vi "GW_update_id.vi"(5 "NULL: workplace_id":i16=-1, 7 "Set null":bool=TRUE, 8 "error in (no error)":errorcluster, 9 "glue_data_id":string="123", 10 "id":i16=5, 11 "DBlink":string="Driver={ODBC Driver 17 for SQL Server};Server=localhost\\SQLEXPRESS;Database=ZDX201;UID=labview;PWD=Dsa@54137926") -> (0 "error out":errorcluster)   [LabVIEW 2019]
uses:
  <vilib>/addons/database/Connection.llb/DB Tools Open Connec (String).vi
  <vilib>/addons/database/Connection.llb/Conn Execute.vi
  <vilib>/addons/database/Recordset.llb/Rec Fetch Recordset Data (R).vi
  <vilib>/addons/database/Recordset.llb/Rec Destroy - Connection.vi
  <vilib>/addons/database/_DB Variant To Data/Database Variant To Data.xnode
  <vilib>/addons/database/NI_Database_API.lvlib
panel:
  out "[glue_workspace]":cluster{"glue_data_id":string}[](array[cluster])
  out "查詢結果":string="Update [workplace_data] \nset  \n[barcode A] = NULL       \n  ,[barcode B] = NULL\n \n  where [workplace_name_id]= -1"
  out "Command":string="where [workplace_name_id]= 5"
  out "update value":T1={"glue_data_id"="123", "update time"=timestamp(3738130170.8632746 s since 1904-01-01)} {"update time" format="%<%.0X %x>T"}
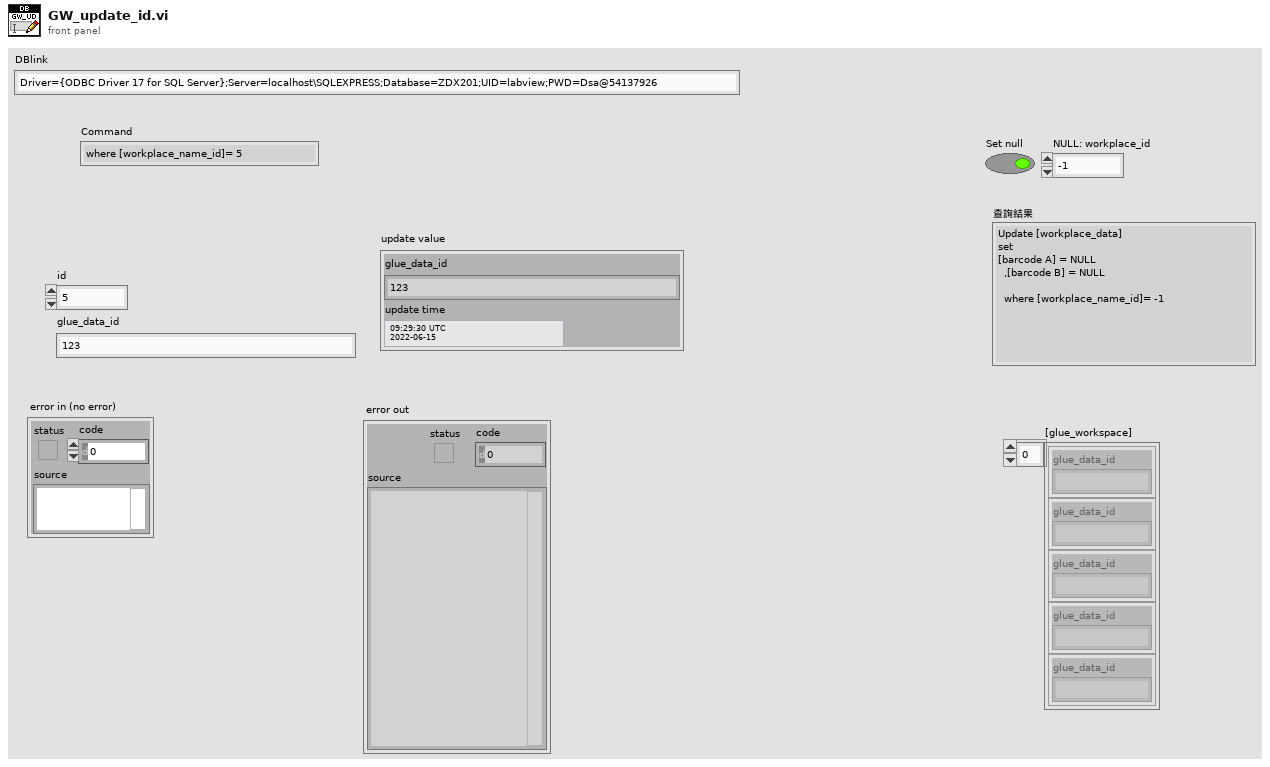
[diagram p1: front panel]
types:
  T1 = cluster{"glue_data_id":string, "update time":timestamp}
  T2 = typedef "NI_Database_API.lvlib/Conn ObjectReference.ctl" = refnum<k1>
  T3 = typedef "NI_Database_API.lvlib/Rec ObjectReference.ctl" = refnum<k1>
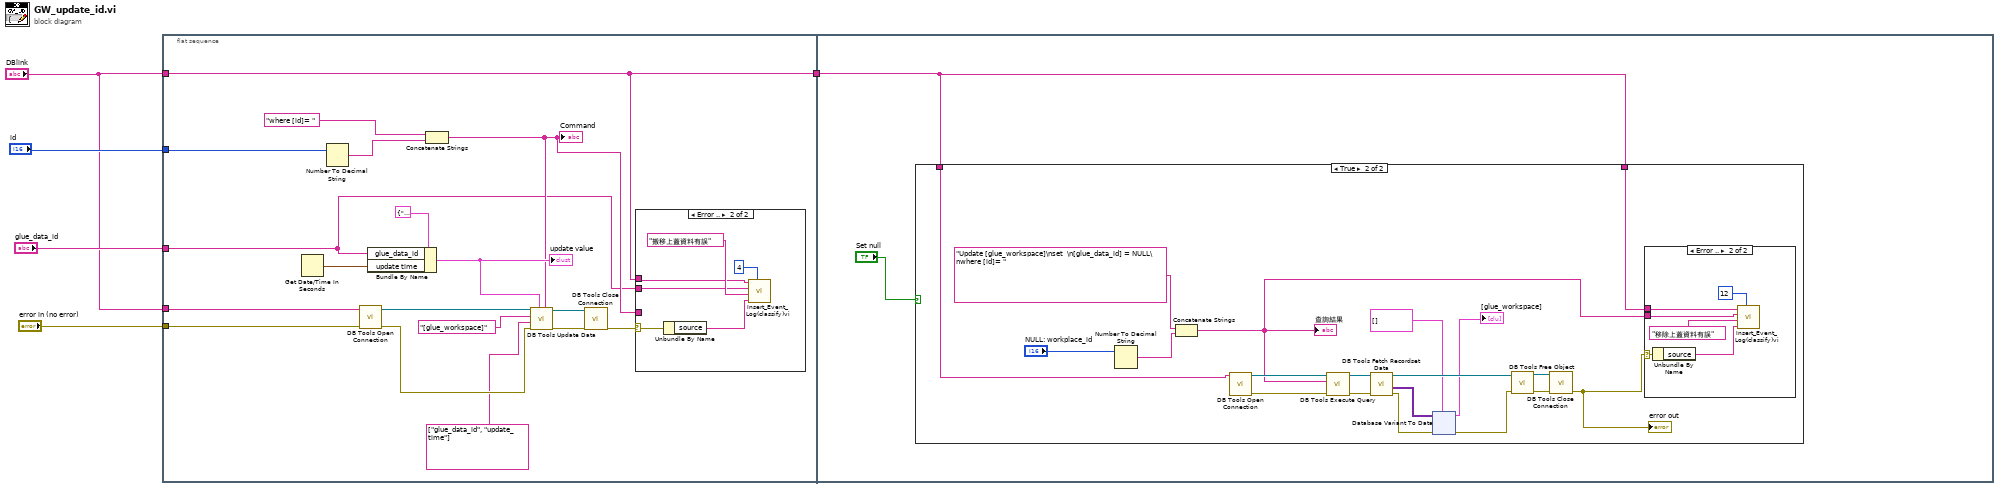
[diagram p0: block diagram]
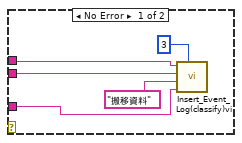
[diagram p2: hidden frame]
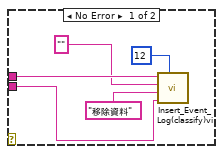
[diagram p4: hidden frame]
diagram:
  n1 = flat-sequence {
    tunnel: "error in (no error)" -> [w23]
    tunnel: "id" -> [w16]
    tunnel: "glue_data_id" -> [w6]
    tunnel: "DBlink" -> [w9]
    tunnel: "DBlink" -> [w7]
    tunnel: [w7] -> w1
    tunnel: w1 -> [w35]
    frame #0 {
      n2 = Get Date/Time In Seconds() -> (seconds since 1Jan1904=w15:timestamp)
      n3 = Number To Decimal String(number=w16) -> (decimal integer string=w13:string)  [unwired: 1 in]
      n4 = call-poly <vilib>:"DB Tools Open Connection.vi"("error in (no error)"=w23, "connection information"=w9) -> ("error out"=w21:errorcluster, "connection reference"=w19:T2)  [unwired: 6 in]
      n5 = Bundle By Name(cluster=T1 {"glue_data_id"="", "update time"=timestamp(0 s since 1904-01-01)} ("update value"), "glue_data_id"=w6, "update time"=w15) -> (w11:T1)
      "update value" <- w11
      n6 = Concatenate Strings("where [id]= ", w13) -> (w8:string)
      "Command" <- w8
      n7 = call <vilib>:"DB Tools Update Data.vi"("condition"=w8, "data"=w11, "error in (no error)"=w21, "columns"=string[] ["glue_data_id", "update_time"], "table"="[glue_workspace]", "connection reference"=w19) -> ("error out"=w22:errorcluster, "connection reference out"=w20:T2)  [unwired: 4 in]
      n8 = call <vilib>:"DB Tools Close Connection.vi"("error in (no error)"=w22, "connection reference"=w20) -> ("error out"=w10:errorcluster)  [unwired: 5 in]
      n9 = case shown="Error .." w10 {
        selector: w10 -> [_ w32]
        tunnel: w8 -> [w25 _]
        tunnel: w7 -> [w26 w30]
        tunnel: w6 -> [w24 w29]
        frame No Error {
          n10 = call "Insert_Event_Log(classify)vi.vi"("classify"=i16 3, "data"=w25, "message"="搬移資料", "id"=w24, "DBlink"=w26) -> ()  [unwired: 6 in, 1 out]
        }
        frame Error {
          n11 = Unbundle By Name(w32) -> ("source"=w31:string)
          n12 = call "Insert_Event_Log(classify)vi.vi"("classify"=i16 4, "data"=w31, "message"="搬移上蓋資料有誤", "id"=w29, "DBlink"=w30) -> ()  [unwired: 6 in, 1 out]
        }
      }
    }
    frame #1 {
      n13 = case shown="True" "Set null" {
        tunnel: w35 -> [_ w39]
        tunnel: w35 -> [_ w38]
        frame False {
        }
        frame True {
          n14 = Number To Decimal String(number="NULL: workplace_id") -> (decimal integer string=w55:string)  [unwired: 1 in]
          n15 = Concatenate Strings("Update [glue_workspace]\nset  \n[glue_data_id] = NULL\nwhere [id]= ", w55) -> (w37:string)
          "查詢結果" <- w37
          n16 = call-poly <vilib>:"DB Tools Open Connection.vi"("connection information"=w39) -> ("error out"=w44:errorcluster, "connection reference"=w45:T2)  [unwired: 7 in]
          n17 = call-poly <vilib>:"DB Tools Execute Query.vi"("error in (no error)"=w44, "SQL query"=w37, "connection reference"=w45) -> ("error out"=w47:errorcluster, "recordset reference"=w46:T3)  [unwired: 5 in]
          n18 = call-poly <vilib>:"DB Tools Fetch Recordset Data.vi"("error in (no error)"=w47, "recordset reference"=w46) -> ("error out"=w52:errorcluster, "recordset data"=w53:variant[][], "recordset reference out"=w51:T3)  [unwired: 3 in]
          n19 = xnode "Database Variant To Data"("database variant"=w53, "error in (no error)"=w52, "type"=cluster{"glue_data_id":string}[] [] ("Workplace: assemble")) -> ("data"=→"[glue_workspace]":cluster{"條碼B":string}[], "error out"=w50:errorcluster)
          n20 = call-poly <vilib>:"DB Tools Free Object.vi"("error in (no error)"=w50, "recordset reference"=w51) -> ("error out"=w49:errorcluster, "connection reference"=w48:T2)  [unwired: 8 in]
          n21 = call <vilib>:"DB Tools Close Connection.vi"("error in (no error)"=w49, "connection reference"=w48) -> ("error out"=w40:errorcluster)  [unwired: 5 in]
          "error out" <- w40
          n22 = case shown="Error .." w40 {
            selector: w40 -> [_ w64]
            tunnel: w38 -> [w58 w62]
            tunnel: w37 -> [w56 w61]
            frame No Error {
              n23 = call "Insert_Event_Log(classify)vi.vi"("classify"=i16 12, "data"=w56, "message"="移除資料", "id"="", "DBlink"=w58) -> ()  [unwired: 6 in, 1 out]
            }
            frame Error {
              n24 = Unbundle By Name(w64) -> ("source"=w63:string)
              n25 = call "Insert_Event_Log(classify)vi.vi"("classify"=i16 12, "data"=w63, "message"="移除上蓋資料有誤", "id"=w61, "DBlink"=w62) -> ()  [unwired: 6 in, 1 out]
            }
          }
        }
      }
    }
  }
